vi "RVC Linear Segment Trajectory.vi"() -> ()   [LabVIEW 2013]
panel:
  out "default velocity":cluster{dbl[], "P(A)":dbl[]}(graph)
  out "default acceleration":cluster{dbl[], "P(A)":dbl[]}(graph)
  out "default position":cluster{dbl[], "P(A)":dbl[]}(graph)
  out "chosen velocity":dbl
  out "velocity":cluster{dbl[], "P(A)":dbl[]}[](graph)
  out "acceleration":cluster{dbl[], "P(A)":dbl[]}[](graph)
  out "position":cluster{dbl[], "P(A)":dbl[]}[](graph)
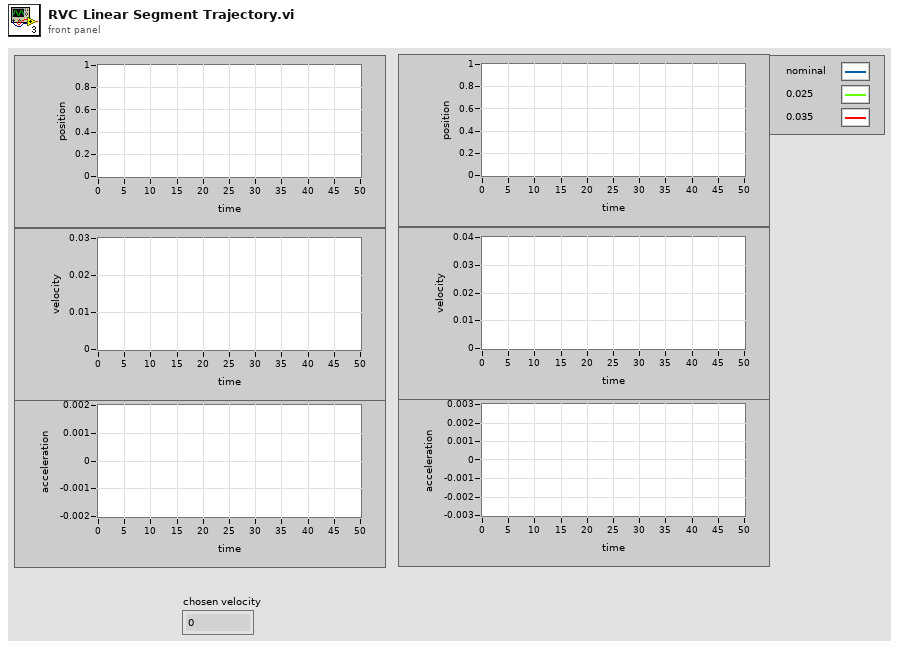
[diagram p1: front panel]
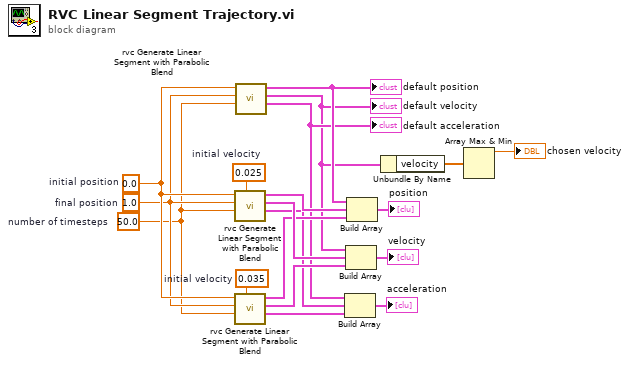
[diagram p0: block diagram]
diagram:
  w15 = 0.035  # initial velocity
  w5 = 50.0  # number of timesteps
  w6 = 1.0  # final position
  w7 = 0.0  # initial position
  w19 = 0.025  # initial velocity
  n1 = call "rvc Generate Linear Segment with Parabolic Blend.vi"("maximum velocity"=w19, "number of timesteps"=w5, "final position"=w6, "initial position"=w7) -> ("acceleration"=w10:cluster{dbl[], "P(A)":dbl[]}, "velocity"=w16:cluster{"time":dbl[], "velocity":dbl[]}, "position"=w12:cluster{"time":dbl[], "position":dbl[]})  [unwired: 4 in, 1 out]
  n2 = call "rvc Generate Linear Segment with Parabolic Blend.vi"("maximum velocity"=w15, "number of timesteps"=w5, "final position"=w6, "initial position"=w7) -> ("acceleration"=w9:cluster{dbl[], "P(A)":dbl[]}, "velocity"=w14:cluster{"time":dbl[], "velocity":dbl[]}, "position"=w11:cluster{"time":dbl[], "position":dbl[]})  [unwired: 4 in, 1 out]
  n3 = call "rvc Generate Linear Segment with Parabolic Blend.vi"("number of timesteps"=w5, "final position"=w6, "initial position"=w7) -> ("acceleration"=w3:cluster{dbl[], "P(A)":dbl[]}, "velocity"=w1:cluster{"time":dbl[], "velocity":dbl[]}, "position"=w4:cluster{"time":dbl[], "position":dbl[]})  [unwired: 5 in, 1 out]
  "default position" <- w4
  "default acceleration" <- w3
  "default velocity" <- w1
  n4 = Build Array(w3, w10, w9) -> (→"acceleration":cluster{dbl[], "P(A)":dbl[]}[])
  n5 = Build Array(w1, w16, w14) -> (→"velocity":cluster{"time":dbl[], "velocity":dbl[]}[])
  n6 = Build Array(w4, w12, w11) -> (→"position":cluster{"time":dbl[], "position":dbl[]}[])
  n7 = Unbundle By Name(w1) -> ("velocity"=w2:dbl[])
  n8 = Array Max & Min(array=w2) -> (max value=→"chosen velocity":dbl)  [unwired: 3 out]
